vi "setup.vi"() -> (2 "Actions":cluster{u32, u32}[](array[cluster]), 3 "Input":cluster{u32, u32}[](array[cluster]))   [LabVIEW 2022 SP3]
panel:
  in  "Actions":cluster{u32, u32}[](array[cluster])
  in  "Input":cluster{u32, u32}[](array[cluster])
  in  "stop":bool
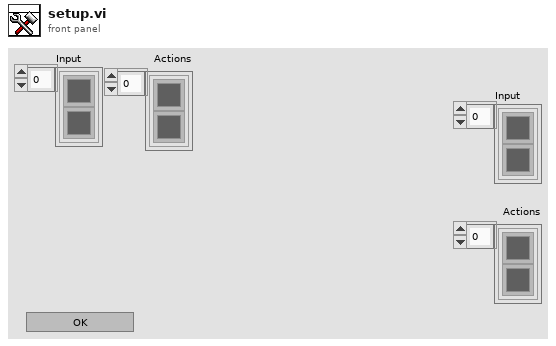
[diagram p1: front panel]
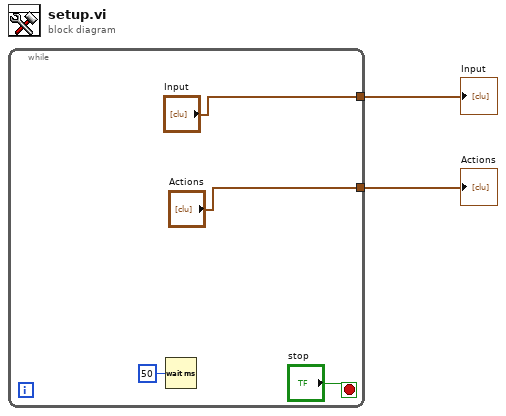
[diagram p0: block diagram]
diagram:
  n1 = while {
    tunnel: ["Input"] -> w2
    tunnel: ["Actions"] -> w1
    stop <- "stop" stop-if-true
    n2 = Wait (ms)(milliseconds to wait=u32 50) -> ()  [unwired: 1 out]
  }
  "Input" <- w2
  "Actions" <- w1
